vi "LoadThresholds.vi"(6 "StationId":u32=1, 8 "error in":errorcluster, 9 "Action (Get)":enum16{"Initialize", "Get"}(ring)=enum."Get", 10 "Index":u32) -> (0 "error out":errorcluster, 1 "Blue or Luma or Val or Inten Range":cluster{"Lower value":i32, "Upper value":i32}, 2 "Green or Sat Range":cluster{"Lower value":i32, "Upper value":i32}, 3 "Red or Hue Range":cluster{"Lower value":i32, "Upper value":i32}, 5 "Color Mode":u16)   [LabVIEW 2018]
uses:
  <vilib>/Utility/config.llb/Read Key (String).vi
  <vilib>/Utility/config.llb/NI_LVConfig.lvlib
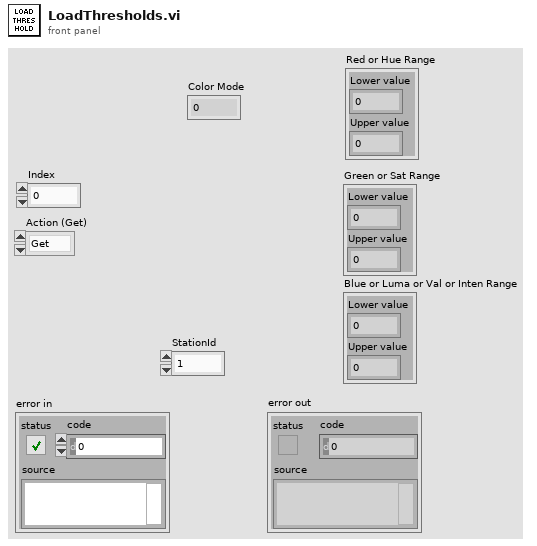
[diagram p1: front panel]
types:
  T1 = typedef "NI_LVConfig.lvlib/Config Data RefNum.ctl" = refnum<k1>
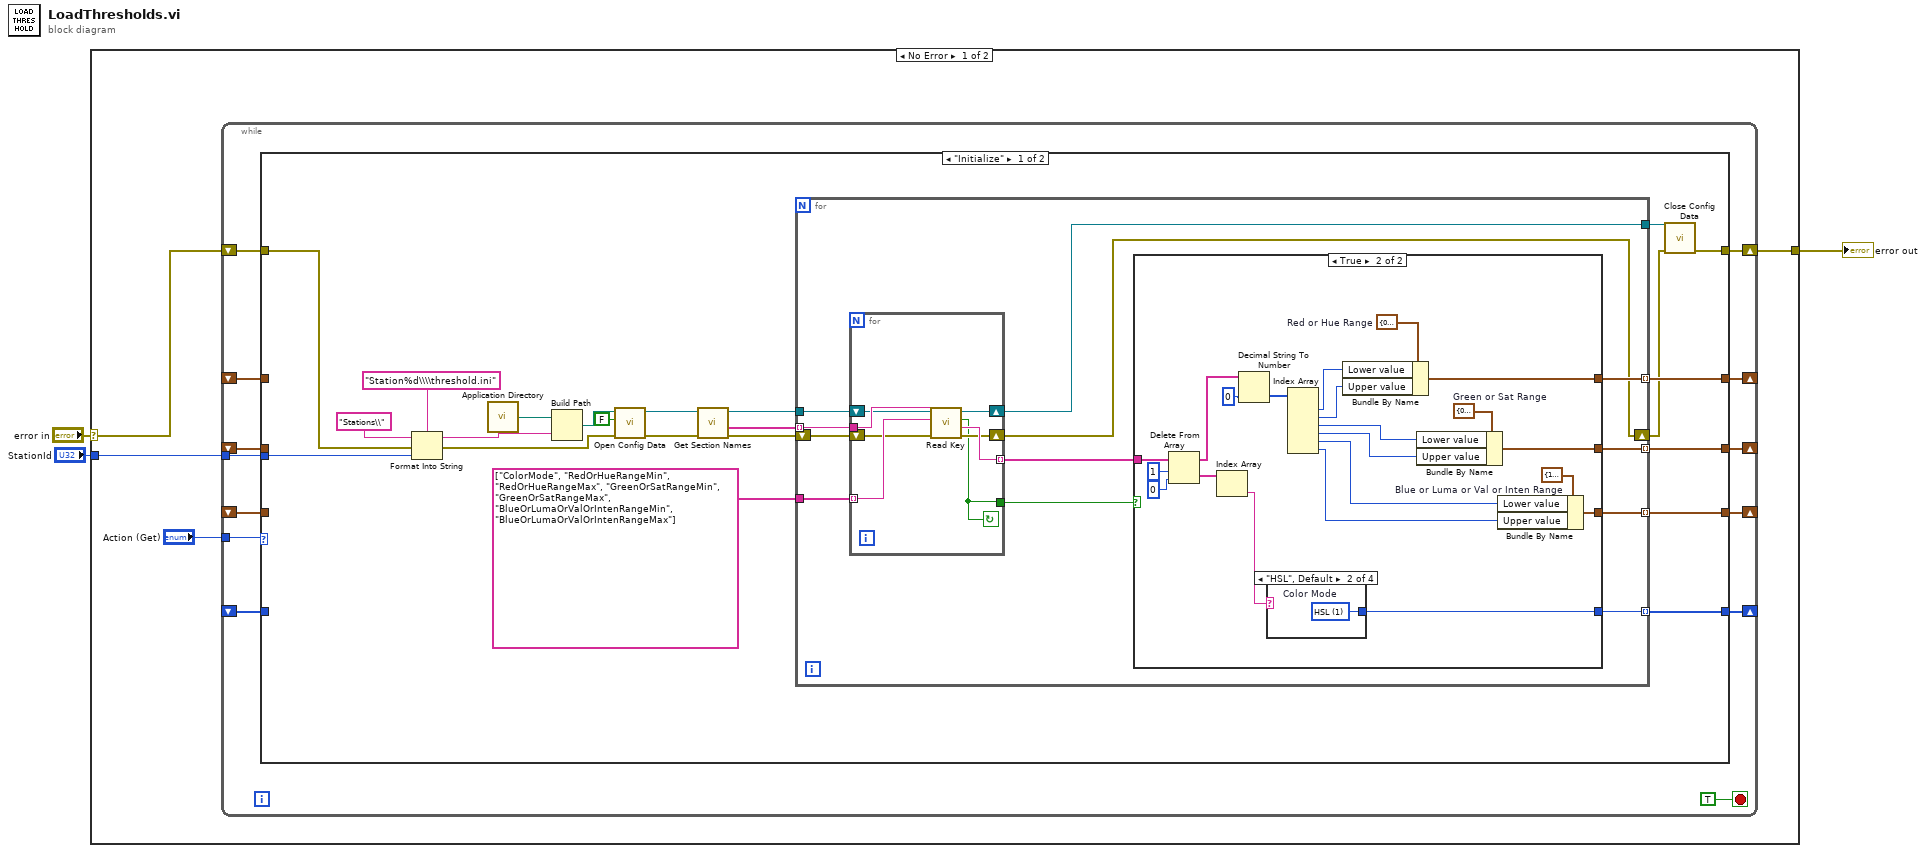
[diagram p0: block diagram]
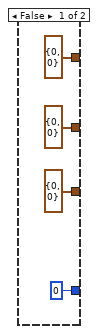
[diagram p2: hidden frame]
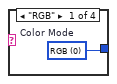
[diagram p3: hidden frame]
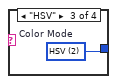
[diagram p4: hidden frame]
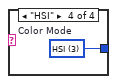
[diagram p5: hidden frame]
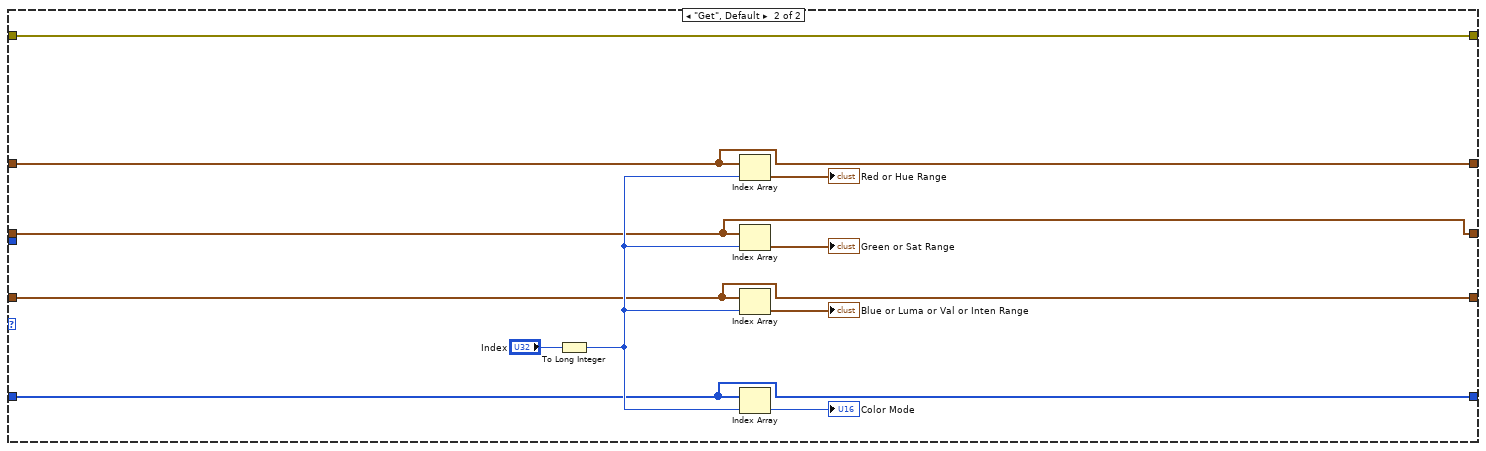
[diagram p6: hidden frame]
diagram:
  n1 = case shown="No Error" "error in" {
    selector: "error in" -> [w6 w103]
    tunnel: "StationId" -> [w7 _]
    tunnel: [w5 w103] -> w1
    frame No Error {
      n2 = while {
        tunnel: w7 -> [w16]
        tunnel: "Action (Get)" -> [w13]
        shift-right: [w14] -> w5
        shift-left: w6 -> [w15]
        shift-right: [w20] -> _
        shift-left: _ -> [w11]
        shift-right: [w19] -> _
        shift-left: _ -> [w10]
        shift-right: [w18] -> _
        shift-left: _ -> [w9]
        shift-right: [w17] -> _
        shift-left: _ -> [w8]
        stop <- TRUE stop-if-true
        n3 = case shown="\"Initialize\"" w13 {
          tunnel: [w37 w95] -> w20
          tunnel: [w36 w94] -> w19
          tunnel: [w35 w93] -> w18
          tunnel: [w34 w92] -> w17
          tunnel: w16 -> [w31 _]
          tunnel: w15 -> [w26 w102]
          tunnel: [w21 w102] -> w14
          tunnel: w11 -> [_ w95]
          tunnel: w10 -> [_ w94]
          tunnel: w9 -> [_ w93]
          tunnel: w8 -> [_ w92]
          frame "Initialize" {
            n4 = Format Into String(format string="Station%d\\\\threshold.ini", initial string="Stations\\", error in=w26, w31) -> (resulting string=w30:string, error out=w28:errorcluster)
            n5 = call <vilib>:"Application Directory.vi"() -> ("Application Directory"=w25:path)
            n6 = Build Path(base path=w25, name or relative path=w30) -> (appended path=w24:path)
            n7 = call <vilib>:"Open Config Data.vi"("error in (no error)"=w28, "create file if necessary (T)"=FALSE, "configuration file path"=w24) -> ("error out"=w41:errorcluster, "refnum"=w42:T1)  [unwired: 6 in, 1 out]
            n8 = call <vilib>:"Get Section Names.vi"("error in (no error)"=w41, "refnum"=w42) -> ("error out"=w27:errorcluster, "section names"=w40:string[], "refnum out"=w39:T1)  [unwired: 7 in]
            n9 = for {
              tunnel: w40 -> [w54] mode=indexing
              tunnel: w39 -> [w53]
              tunnel: string[] ["ColorMode", "RedOrHueRangeMin", "RedOrHueRangeMax", "GreenOrSatRangeMin", "GreenOrSatRangeMax", "BlueOrLumaOrValOrIntenRangeMin", "BlueOrLumaOrValOrIntenRangeMax"] -> [w52]
              tunnel: [w50] -> w37 mode=indexing
              tunnel: [w49] -> w36 mode=indexing
              tunnel: [w48] -> w35 mode=indexing
              tunnel: [w47] -> w34 mode=indexing
              shift-right: [w44] -> w22
              shift-left: w27 -> [w46]
              tunnel: [w43] -> w23
              n10 = for {
                tunnel: w54 -> [w91]
                tunnel: w52 -> [w89] mode=indexing
                tunnel: [w88] -> w51 mode=indexing
                shift-right: [w86] -> w44
                shift-left: w46 -> [w87]
                shift-right: [w85] -> w43
                shift-left: w53 -> [w90]
                tunnel: [w84] -> w45
                stop <- w84 continue-if-true
                n11 = call-poly <vilib>:"Read Key.vi"("section"=w91, "error in (no error)"=w87, "key"=w89, "refnum"=w90) -> ("error out"=w86:errorcluster, "value"=w88:string, "found?"=w84:bool, "refnum out"=w85:T1)  [unwired: 4 in]
              }
              n12 = case shown="True" w45 {
                tunnel: w51 -> [_ w79]
                tunnel: [cluster{"Lower value":i32, "Upper value":i32} {"Lower value"=0, "Upper value"=0} ("Red or Hue Range") w62] -> w50
                tunnel: [cluster{"Lower value":i32, "Upper value":i32} {"Lower value"=0, "Upper value"=0} ("Green or Sat Range") w61] -> w49
                tunnel: [cluster{"Lower value":i32, "Upper value":i32} {"Lower value"=0, "Upper value"=0} ("Blue or Luma or Val or Inten Range") w60] -> w48
                tunnel: [u16 0 ("Color Mode") w59] -> w47
                frame False {
                }
                frame True {
                  w65 = cluster{"Lower value":i32, "Upper value":i32} {"Lower value"=143, "Upper value"=248}  # Blue or Luma or Val or Inten Range
                  w70 = cluster{"Lower value":i32, "Upper value":i32} {"Lower value"=0, "Upper value"=17}  # Green or Sat Range
                  w71 = cluster{"Lower value":i32, "Upper value":i32} {"Lower value"=0, "Upper value"=255}  # Red or Hue Range
                  n13 = Delete From Array(array=w79, length=1, index=0) -> (deleted portion=w76:string[], array with subset deleted=w74:string[])
                  n14 = Index Array(array=w76) -> (element=w75:string)  [unwired: 1 in]
                  n15 = Decimal String To Number(string=w74, default (0L)=0 ("default (0 I32)")) -> (number=w72:i32[])  [unwired: 1 in, 1 out]
                  n16 = case shown="\"HSL\", Default" w75 {
                    tunnel: [w80 w81 w82 w83] -> w59
                    frame "RGB" {
                      w80 = u16 0 items=["RGB", "HSL", "HSV", "HSI"]  # Color Mode
                    }
                    frame "HSL", Default {
                      w81 = u16 1 items=["RGB", "HSL", "HSV", "HSI"]  # Color Mode
                    }
                    frame "HSV" {
                      w82 = u16 2 items=["RGB", "HSL", "HSV", "HSI"]  # Color Mode
                    }
                    frame "HSI" {
                      w83 = u16 3 items=["RGB", "HSL", "HSV", "HSI"]  # Color Mode
                    }
                  }
                  n17 = Index Array(array=w72) -> (element #1=w69:i32, element #2=w68:i32, element #3=w67:i32, element #4=w66:i32, element #5=w64:i32, element #6=w63:i32)  [unwired: 6 in]
                  n18 = Bundle By Name(cluster=w71, "Lower value"=w69, "Upper value"=w68) -> (w62:cluster{"Lower value":i32, "Upper value":i32})
                  n19 = Bundle By Name(cluster=w70, "Lower value"=w67, "Upper value"=w66) -> (w61:cluster{"Lower value":i32, "Upper value":i32})
                  n20 = Bundle By Name(cluster=w65, "Lower value"=w64, "Upper value"=w63) -> (w60:cluster{"Lower value":i32, "Upper value":i32})
                }
              }
            }
            n21 = call <vilib>:"Close Config Data.vi"("error in (no error)"=w22, "refnum"=w23) -> ("error out"=w21:errorcluster)  [unwired: 8 in, 1 out]
          }
          frame "Get", Default {
            n22 = To Long Integer(number="Index") -> (32bit integer=w96:i32)
            n23 = Index Array(array=w95, index=w96) -> (element=→"Red or Hue Range":cluster{"Lower value":i32, "Upper value":i32})
            n24 = Index Array(array=w94, index=w96) -> (element=→"Green or Sat Range":cluster{"Lower value":i32, "Upper value":i32})
            n25 = Index Array(array=w93, index=w96) -> (element=→"Blue or Luma or Val or Inten Range":cluster{"Lower value":i32, "Upper value":i32})
            n26 = Index Array(array=w92, index=w96) -> (element=→"Color Mode":u16)
          }
        }
      }
    }
    frame Error {
    }
  }
  "error out" <- w1
